vi "Deg to Rad 1D(dbl).vi"(1 "degrees":dbl[](array[numeric]) format="%.2f") -> (0 "radians":dbl[](array[numeric]) format="%.2f")   [LabVIEW 2012, in "几何工具.lvlib"]
doc: "功能：\n\n一维数组角度转换为弧度。\n\n输入：角度，单位为度。\n\n输出：弧度。\n\ncsxcs_366创建。"
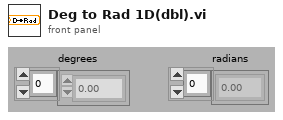
[diagram p1: front panel]
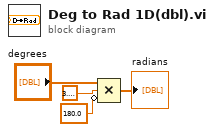
[diagram p0: block diagram]
diagram:
  n1 = Compound Arithmetic op=MULTIPLY("degrees", 3.141592653589793, invert 180.0 ("值")) -> (→"radians":dbl[])
